vi "TemplateModule.CreateRequests.vi"(8 "error in (no error)":errorcluster) -> (0 "error out":errorcluster, 3 "Requests":T1)   [LabVIEW 2024, in "TemplateModule.lvclass"]
uses:
  TemplateModule.lvclass
  Request Events--cluster.ctl
  Do Something Args.ctl
  RQMHCore/ModuleCore/Reply.ctl
  JamesT Args.ctl
  RRRR Args.ctl
   Args.ctl
  RQMHCore/ModuleCore/RQMHModule.lvclass
  test Args.ctl
  testering Args.ctl
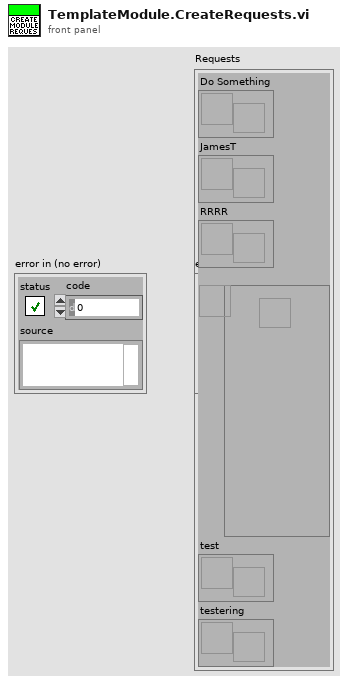
[diagram p1: front panel]
types:
  T1 = typedef "TemplateModule.lvclass/Request Events--cluster.ctl" = cluster{"Do Something":refnum<user-event>, "JamesT":refnum<user-event>, "RRRR":refnum<user-event>, refnum<user-event>, "test":refnum<user-event>, "testering":refnum<user-event>}
  T2 = typedef "TemplateModule.lvclass/testering Args.ctl" = cluster{"RQMHModule.lvclass":refnum<class "RQMHModule.lvclass">}
  T3 = typedef "RQMHModule.lvclass/Reply.ctl" = cluster{"Expects Reply":bool, "Reply":refnum<notifier>}
  T4 = typedef "TemplateModule.lvclass/test Args.ctl" = cluster{"String":string}
  T5 = typedef "TemplateModule.lvclass/JamesT Args.ctl" = cluster{"Boolean":bool}
  T6 = typedef "TemplateModule.lvclass/Do Something Args.ctl" = cluster{"Msg":string}
  T7 = cluster{"Do Something Args":T6, "Reply Payload":T3}
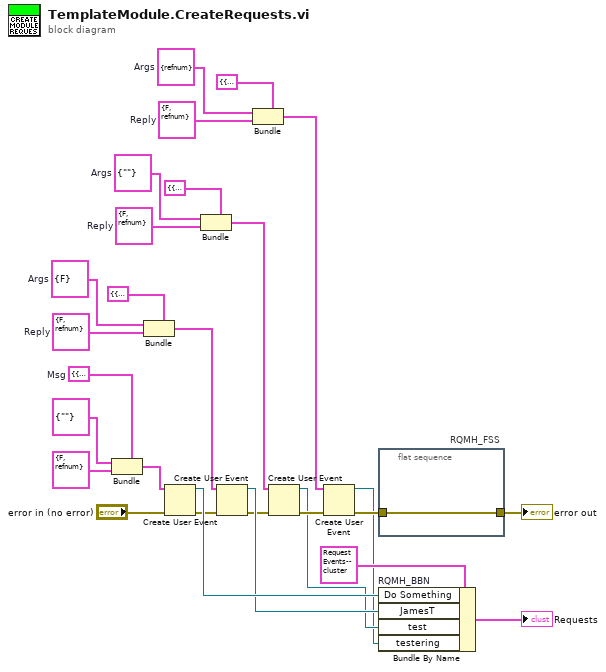
[diagram p0: block diagram]
diagram:
  w4 = T2 {"RQMHModule.lvclass"=refnum}  # Args
  w3 = T3 {"Expects Reply"=FALSE, "Reply"=refnum}  # Reply
  w10 = T4 {"String"=""}  # Args
  w9 = T3 {"Expects Reply"=FALSE, "Reply"=refnum}  # Reply
  w19 = T5 {"Boolean"=FALSE}  # Args
  w18 = T3 {"Expects Reply"=FALSE, "Reply"=refnum}  # Reply
  w22 = T7 {"Do Something Args"={"Msg"=""}, "Reply Payload"={"Expects Reply"=FALSE, "Reply"=refnum}}  # Msg
  n1 = Bundle(cluster=w22, "Do Something Args"=T6 {"Msg"=""}, "Reply Payload"=T3 {"Expects Reply"=FALSE, "Reply"=refnum}) -> (w25:T7)
  n2 = Bundle(cluster=cluster{"Args":T5, "Reply":T3} {"Args"={"Boolean"=FALSE}, "Reply"={"Expects Reply"=FALSE, "Reply"=refnum}} ("Msg"), "Args"=w19, "Reply"=w18) -> (w17:cluster{"Args":T5, "Reply":T3})
  n3 = Create User Event(user event datatype=w25, error in="error in (no error)") -> (user event=w21:refnum<user-event>, error out=w15:errorcluster)
  n4 = Bundle(cluster=cluster{"Args":T4, "Reply":T3} {"Args"={"String"=""}, "Reply"={"Expects Reply"=FALSE, "Reply"=refnum}} ("Msg"), "Args"=w10, "Reply"=w9) -> (w8:cluster{"Args":T4, "Reply":T3})
  n5 = Create User Event(user event datatype=w17, error in=w15) -> (user event=w14:refnum<user-event>, error out=w13:errorcluster)
  n6 = Bundle(cluster=cluster{"Args":T2, "Reply":T3} {"Args"={"RQMHModule.lvclass"=refnum}, "Reply"={"Expects Reply"=FALSE, "Reply"=refnum}} ("Msg"), "Args"=w4, "Reply"=w3) -> (w2:cluster{"Args":T2, "Reply":T3})
  n7 = Create User Event(user event datatype=w8, error in=w13) -> (user event=w11:refnum<user-event>, error out=w12:errorcluster)
  n8 = Create User Event(user event datatype=w2, error in=w12) -> (user event=w5:refnum<user-event>, error out=w6:errorcluster)
  n9 = flat-sequence "RQMH_FSS" {
    tunnel: [w29] -> w20
    tunnel: w6 -> [w29]
    frame #0 {
    }
  }
  n10 = Bundle By Name "RQMH_BBN"(cluster=T1 {"Do Something"=refnum, "JamesT"=refnum, "RRRR"=refnum, "User Event"=refnum, "test"=refnum, "testering"=refnum} ("Requests"), "Do Something"=w21, "JamesT"=w14, "test"=w11, "testering"=w5) -> (→"Requests":T1)
  "error out" <- w20
